vi "ColorGraphMarkers_LS1.vi"(8 "error in (no error)":errorcluster caption="entrée d'erreur (pas d'erreur)", 9 "DataMin":dbl, 10 "DataMax":dbl, 11 "GraphRef":refnum<vi>) -> (0 "error out":errorcluster caption="sortie d'erreur", 1 "MarkersOut":cluster{dbl, u32}[](array[cluster]))   [LabVIEW 2019]
doc: "Utilisez ce modèle pour construire un VI à utiliser en tant que sous-VI."
panel:
  out "MarkersIn":cluster{dbl, u32}[](array[cluster])
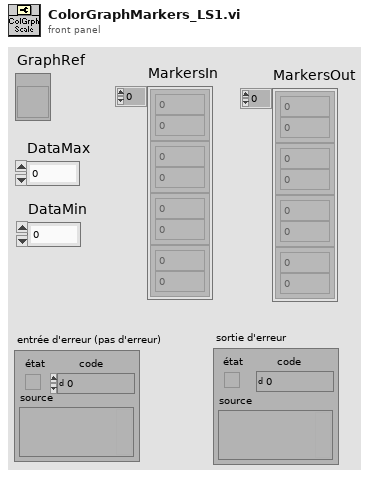
[diagram p1: front panel]
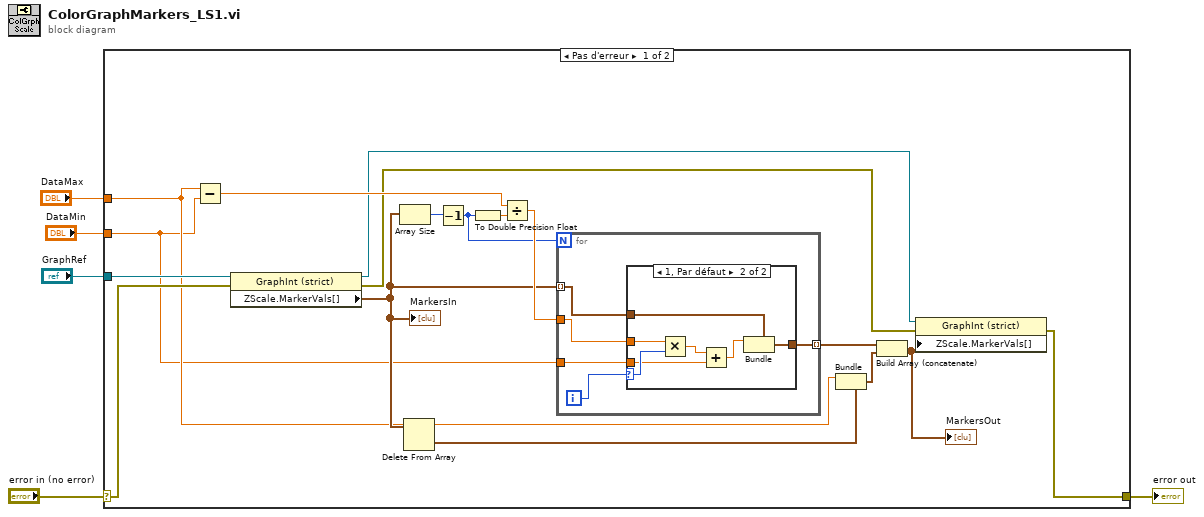
[diagram p0: block diagram]
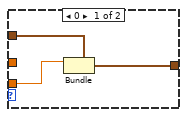
[diagram p2: hidden frame]
diagram:
  n1 = case shown="Pas d'erreur" "error in (no error)" {
    selector: "error in (no error)" -> [w10 w38]
    tunnel: [w8 w38] -> w4
    tunnel: "GraphRef" -> [w22 _]
    tunnel: "DataMin" -> [w6 _]
    tunnel: "DataMax" -> [w7 _]
    frame No Error {
      n2 = Subtract(x=w7, y=w6) -> (x-y=w21:dbl)
      n3 = property on="Nœud de propriété" class="GraphInt (strict)"(reference=w22, error in=w10) -> (reference out=w11:refnum<vi>, error out=w9:errorcluster, "ZScale.MarkerVals[]"=w15:cluster{dbl, u32}[])
      "MarkersIn" <- w15
      n4 = Array Size(array=w15) -> (size(s)=w19:i32)
      n5 = Delete From Array(array=w15) -> (deleted portion=w12:cluster{dbl, u32})  [unwired: 2 in, 1 out]
      n6 = Decrement(x=w19) -> (x-1=w16:i32)
      n7 = To Double Precision Float(number=w16) -> (double precision float=w20:dbl)
      n8 = Divide(x=w21, y=w20) -> (x/y=w18:dbl)
      n9 = for {
        N: w16 -> [_]
        tunnel: w6 -> [w25]
        tunnel: w18 -> [w23]
        tunnel: w15 -> [w26] mode=indexing
        tunnel: [w24] -> w17 mode=indexing
        i -> [w27]
        n10 = case shown="1, Par défaut" w27 {
          selector: w27 -> [_ w36]
          tunnel: w26 -> [w30 w33]
          tunnel: w25 -> [w29 w34]
          tunnel: [w28 w32] -> w24
          tunnel: w23 -> [_ w37]
          frame 0 {
            n11 = Bundle(cluster=w30, w29) -> (w28:cluster{dbl, u32})  [unwired: 1 in]
          }
          frame 1, Default {
            n12 = Multiply(x=w37, y=w36) -> (x*y=w35:dbl)
            n13 = Add(x=w35, y=w34) -> (x+y=w31:dbl)
            n14 = Bundle(cluster=w33, w31) -> (w32:cluster{dbl, u32})  [unwired: 1 in]
          }
        }
      }
      n15 = Bundle(cluster=w12, w7) -> (w13:cluster{dbl, u32})  [unwired: 1 in]
      n16 = Build Array (concatenate)(w17, w13) -> (w14:cluster{dbl, u32}[])
      "MarkersOut" <- w14
      n17 = property on="Nœud de propriété" class="GraphInt (strict)"(reference=w11, error in=w9, "ZScale.MarkerVals[]"=w14) -> (error out=w8:errorcluster)  [unwired: 1 out]
    }
    frame Error {
    }
  }
  "error out" <- w4
